vi "GEN2_Read_Pack.vi"(8 "error in (no error)":errorcluster, 11 "VISA Refnum in":refnum<visa-resource-name>) -> (0 "error out":errorcluster, 2 "Pack data":T1, 3 "VISA Refnum out":refnum<visa-resource-name>)   [LabVIEW 2016, in "GEN_2.lvlib"]
uses:
  GEN_2.lvlib
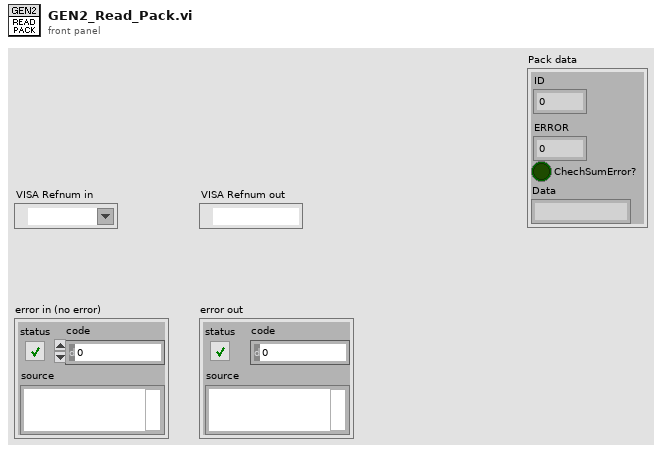
[diagram p1: front panel]
types:
  T1 = cluster{"ID":u8, "ERROR":u8, "ChechSumError?":bool, "Data":string}
  T2 = enum16{"big-endian, network order", "native, host order", "little-endian"}
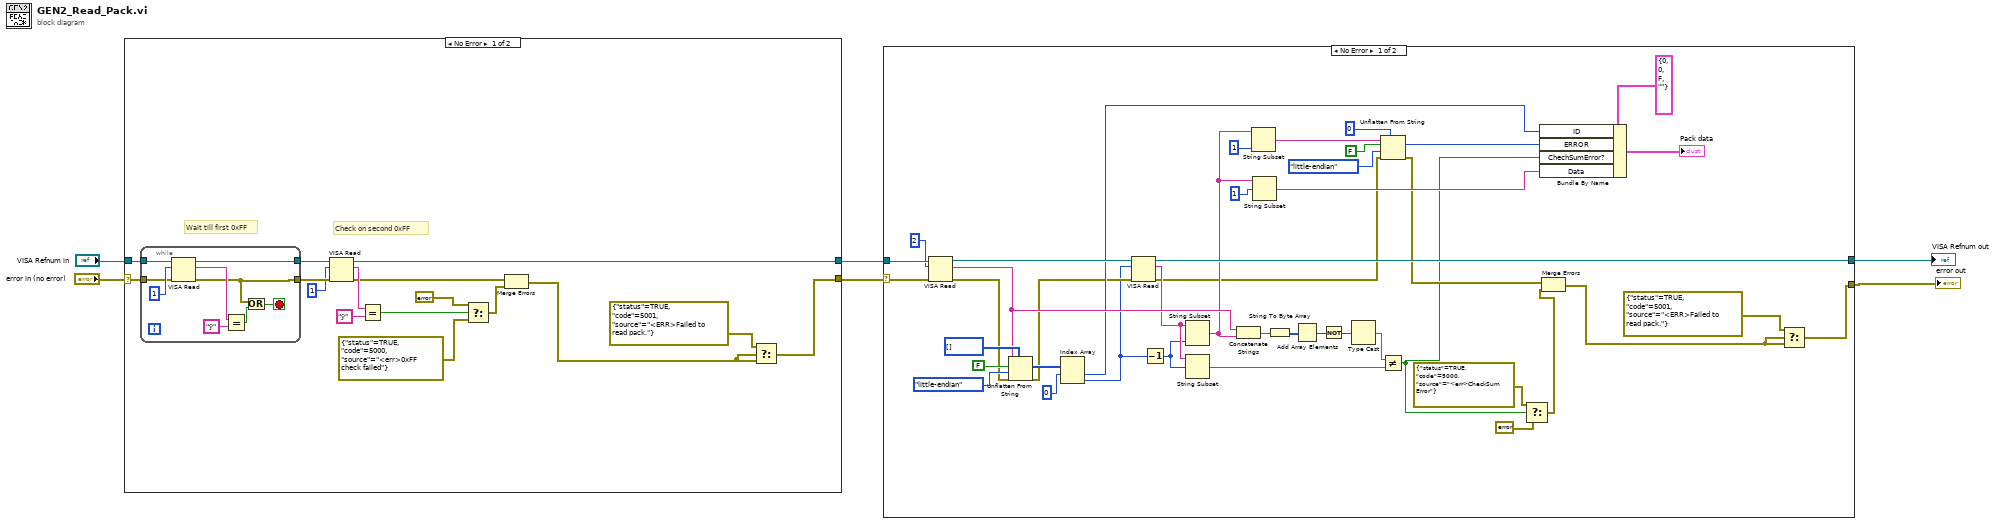
[diagram p0: block diagram]
diagram:
  n1 = case shown="No Error" "error in (no error)" {
    selector: "error in (no error)" -> [w11 w32]
    tunnel: [w22 w33] -> w4
    tunnel: "VISA Refnum in" -> [w19 w33]
    tunnel: [w9 w32] -> w2
    frame No Error {
      # "Check on second 0xFF"
      # "Wait till first 0xFF"
      n2 = while {
        tunnel: [w23] -> w21
        tunnel: w11 -> [w27]
        tunnel: w19 -> [w26]
        tunnel: [w25] -> w20
        stop <- w28 stop-if-true
        n3 = VISA Read(VISA resource name=w26, byte count=u32 1, error in (no error)=w27) -> (VISA resource name out=w25:refnum<visa-resource-name>, read buffer=w30:string, error out=w23:errorcluster)  [unwired: 1 out]
        n4 = Equal?(x=w30, y="ÿ") -> (x = y?=w24:bool)
        n5 = Or(x=w23, y=w24) -> (x .or. y?=w28:bool)
      }
      n6 = VISA Read(VISA resource name=w20, byte count=u32 1, error in (no error)=w21) -> (VISA resource name out=w22:refnum<visa-resource-name>, read buffer=w17:string, error out=w13:errorcluster)  [unwired: 1 out]
      n7 = Equal?(x=w17, y="ÿ") -> (x = y?=w15:bool)
      n8 = Select(t=errorcluster {"status"=FALSE, "code"=0, "source"=""} ("No Error"), s=w15, f=errorcluster {"status"=TRUE, "code"=5000, "source"="<err>0xFF check failed"} ("FF")) -> (s? t:f=w12:errorcluster)
      n9 = Merge Errors(w13, w12) -> (w7:errorcluster)
      n10 = Select(t=errorcluster {"status"=TRUE, "code"=5001, "source"="<ERR>Failed to read pack."} ("5001"), s=w7, f=w7) -> (s? t:f=w9:errorcluster)
    }
    frame Error {
    }
  }
  n11 = case shown="No Error" w2 {
    selector: w2 -> [w67 w77]
    tunnel: [w76 w78] -> w6
    tunnel: [w38 w77] -> w5
    tunnel: w4 -> [w69 w78]
    frame No Error {
      n12 = VISA Read(VISA resource name=w69, byte count=u32 2, error in (no error)=w67) -> (VISA resource name out=w73:refnum<visa-resource-name>, read buffer=w66:string, error out=w46:errorcluster)  [unwired: 1 out]
      n13 = Unflatten From String(type=u8[] [], binary string=w66, data includes array or string size? (T)=FALSE, byte order (0:big-endian, network order)=T2."little-endian", error in (no error)=w46) -> (value=w74:u8[], error out=w45:errorcluster)  [unwired: 1 out]
      n14 = Index Array(array=w74, index #1=0 ("index")) -> (element #1=w49:u8, element #2=w44:u8)  [unwired: 1 in]
      n15 = VISA Read(VISA resource name=w73, byte count=w44, error in (no error)=w45) -> (VISA resource name out=w76:refnum<visa-resource-name>, read buffer=w61:string, error out=w42:errorcluster)  [unwired: 1 out]
      n16 = Decrement(x=w44) -> (x-1=w43:u8)
      n17 = String Subset(string=w61, length (rest)=w43) -> (substring=w56:string)  [unwired: 1 in]
      n18 = String Subset(string=w61, offset (0)=w43) -> (substring=w60:string)  [unwired: 1 in]
      n19 = Concatenate Strings(w66, w56) -> (w63:string)
      n20 = String Subset(string=w56, length (rest)=u8 1 ("y")) -> (substring=w53:string)  [unwired: 1 in]
      n21 = String Subset(string=w56, offset (0)=u8 1 ("y")) -> (substring=w47:string)  [unwired: 1 in]
      n22 = String To Byte Array(string=w63) -> (unsigned byte array=w64:u8[])
      n23 = Add Array Elements(numeric array=w64) -> (sum=w65:u8)
      n24 = Not(x=w65) -> (.not. x?=w62:u8)
      n25 = Type Cast(x=w62) -> (*(type *) &x=w59:string)  [unwired: 1 in]
      n26 = Unflatten From String(type=u8 0 ("y"), binary string=w53, data includes array or string size? (T)=FALSE, byte order (0:big-endian, network order)=T2."little-endian", error in (no error)=w42) -> (value=w51:u8, error out=w41:errorcluster)  [unwired: 1 out]
      n27 = Not Equal?(x=w59, y=w60) -> (x != y?=w40:bool)
      n28 = Select(t=errorcluster {"status"=TRUE, "code"=5000, "source"="<err>CheckSum Error"} ("FF"), s=w40, f=errorcluster {"status"=FALSE, "code"=0, "source"=""}) -> (s? t:f=w39:errorcluster)
      n29 = Bundle By Name(cluster=T1 {"ID"=0, "ERROR"=0, "ChechSumError?"=FALSE, "Data"=""} ("output cluster"), "ID"=w49, "ERROR"=w51, "ChechSumError?"=w40, "Data"=w47) -> (→"Pack data":T1)
      n30 = Merge Errors(w41, w39) -> (w37:errorcluster)
      n31 = Select(t=errorcluster {"status"=TRUE, "code"=5001, "source"="<ERR>Failed to read pack."} ("5001"), s=w37, f=w37) -> (s? t:f=w38:errorcluster)
    }
    frame Error {
    }
  }
  "VISA Refnum out" <- w6
  "error out" <- w5
